vi "ke37xx Time and Date.vi"(0 "VISA Resource Name":refnum<visa-resource-name>, 7 "Time and Date Value":timestamp format="%<%H:%M:%S\n%Y/%m/%d>T", 11 "error in (no error)":errorcluster) -> (4 "VISA Resource Name Out":refnum<visa-resource-name>, 15 "error out":errorcluster)   [LabVIEW 2009, in "Keithley 3700 Series.lvlib"]
doc: "Use this VI to set the current Time and Date on your instrument."
uses:
  <instrlib>/Keithley 3706/Keithley 3700 Series.lvlib
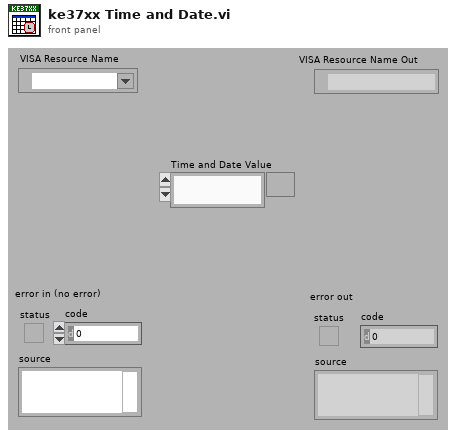
[diagram p1: front panel]
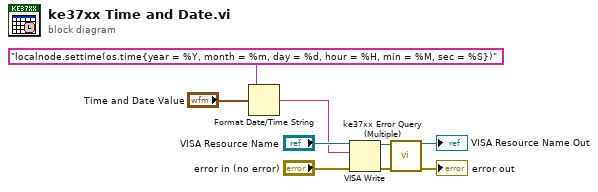
[diagram p0: block diagram]
diagram:
  n1 = Format Date/Time String(time format string (%c)="localnode.settime(os.time{year = %Y, month = %m, day = %d, hour = %H, min = %M, sec = %S})" ("format string"), seconds (now)="Time and Date Value") -> (date/time string=w1:string)  [unwired: 1 out]
  n2 = VISA Write(VISA resource name="VISA Resource Name", write buffer=w1, error in (no error)="error in (no error)") -> (VISA resource name out=w5:refnum<visa-resource-name>, error out=w4:errorcluster)  [unwired: 1 out]
  n3 = call <instrlib>:"ke37xx Error Query (Multiple).vi"("VISA resource name"=w5, "error in (no error)"=w4) -> ("VISA resource name out"=→"VISA Resource Name Out":refnum<visa-resource-name>, "error out"=→"error out":errorcluster)  [unwired: 12 out]
